vi "Shaker_DAQ.vi"() -> ()   [LabVIEW 2015]
uses:
  <vilib>/express/express analysis/Spectral/Block/exnSpectralBlock spectral measurements RMS poly.vi
  <vilib>/express/express analysis/Spectral/Block/exnSpectralBlock spectral measurements RMS DDT.vi
  <vilib>/express/express analysis/Spectral/XNode/ExpressSpectralMeasurementsBlockNode.xnode
panel:
  in  "Tab Control":T1(tab)
  in  "Test Folder":string
  in  "Input Signal":string(combo)
  in  "Date":string
  in  "PCB Type":string(combo)
  out "Beam Acceleration":dynamicdata(graph)
  out "FRF":dynamicdata(graph)
  out "FFT Magnitude":dynamicdata(graph)
  out "FFT Phase":dynamicdata(graph)
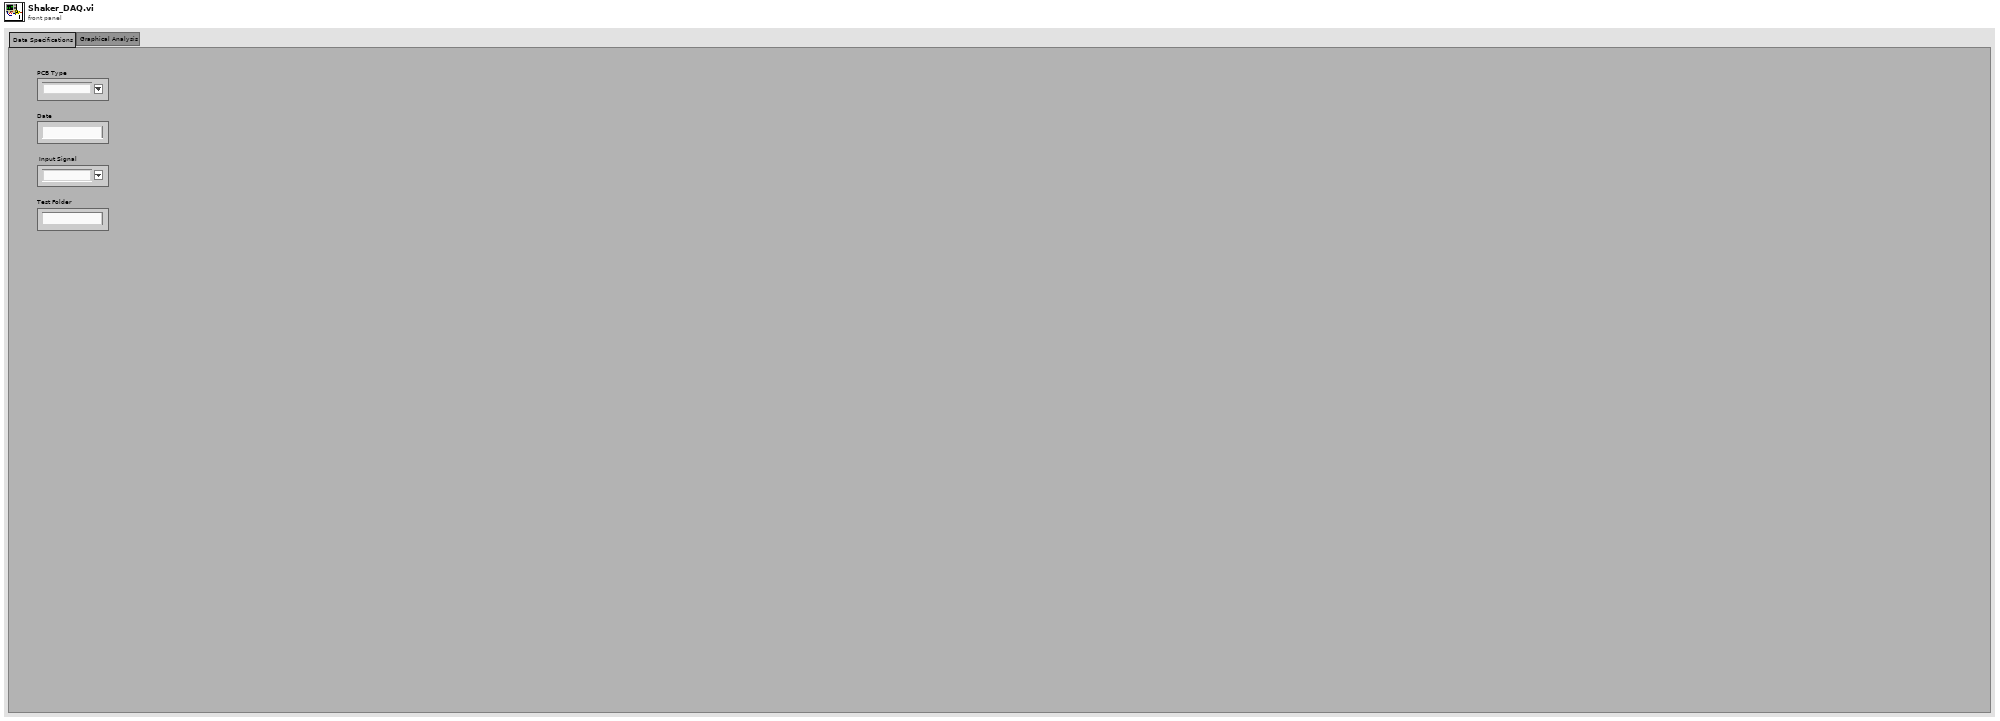
[diagram p1: front panel]
types:
  T1 = enum32{"Data Specifications", "Graphical Analysis"}
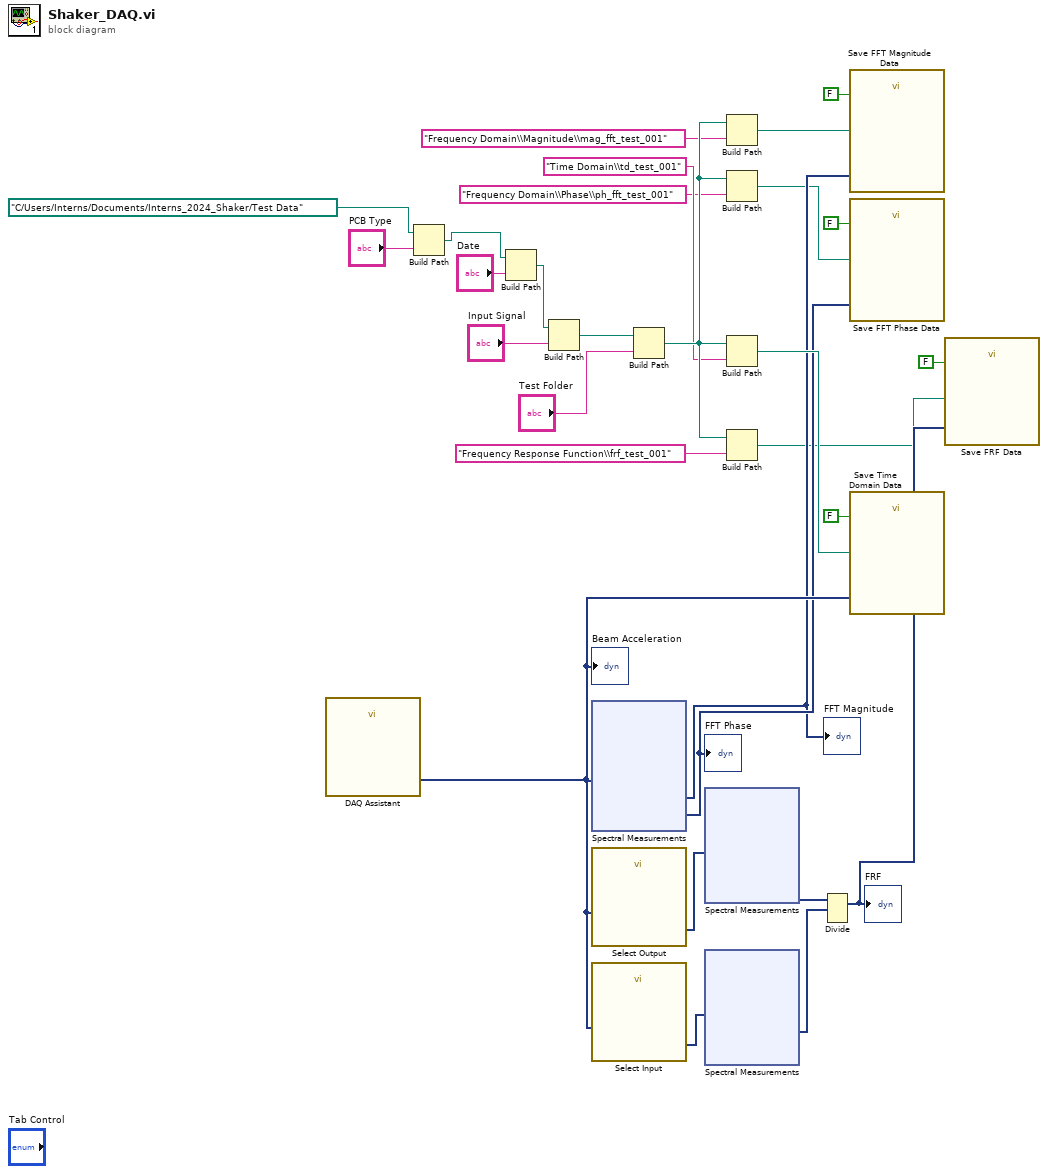
[diagram p0: block diagram]
diagram:
  n1 = call "DAQ Assistant"() -> ("data"=w10:dynamicdata)  [unwired: 17 in, 2 out]
  "Beam Acceleration" <- w10
  n2 = Build Path(base path=path "C:/Users/Interns/Documents/Interns_2024_Shaker/Test Data", name or relative path="PCB Type") -> (appended path=w24:path)
  n3 = Build Path(base path=w24, name or relative path="Date") -> (appended path=w19:path)
  n4 = Build Path(base path=w19, name or relative path="Input Signal") -> (appended path=w18:path)
  n5 = xnode "Spectral Measurements"("Signals"=w10) -> ("FFT - (RMS)"=w8:dynamicdata, "Phase"=w9:dynamicdata)  [unwired: 1 in, 1 out]
  "FFT Magnitude" <- w8
  "FFT Phase" <- w9
  n6 = call "Select Output"("Signals"=w10) -> ("Signal Out"=w26:dynamicdata)  [unwired: 9 in, 1 out]
  n7 = call "Select Input"("Signals"=w10) -> ("Signal Out"=w27:dynamicdata)  [unwired: 9 in, 1 out]
  n8 = Build Path(base path=w18, name or relative path="Test Folder") -> (appended path=w12:path)
  n9 = xnode "Spectral Measurements"("Signals"=w26) -> ("FFT - (RMS)"=w28:dynamicdata)  [unwired: 1 in, 2 out]
  n10 = xnode "Spectral Measurements"("Signals"=w27) -> ("FFT - (RMS)"=w29:dynamicdata)  [unwired: 1 in, 2 out]
  n11 = Build Path(base path=w12, name or relative path="Frequency Domain\\Magnitude\\mag_fft_test_001") -> (appended path=w3:path)
  n12 = Build Path(base path=w12, name or relative path="Frequency Domain\\Phase\\ph_fft_test_001") -> (appended path=w6:path)
  n13 = Build Path(base path=w12, name or relative path="Time Domain\\td_test_001") -> (appended path=w11:path)
  n14 = Build Path(base path=w12, name or relative path="Frequency Response Function\\frf_test_001") -> (appended path=w2:path)
  n15 = Divide(1:w29, 2:w28) -> (0:w13:dynamicdata)  [unwired: 1 in, 1 out]
  "FRF" <- w13
  n16 = call "Save FFT Magnitude Data"("Signals"=w8, "Enable"=FALSE, "Filename"=w3) -> ()  [unwired: 14 in, 3 out]
  n17 = call "Save FFT Phase Data"("Signals"=w9, "Enable"=FALSE, "Filename"=w6) -> ()  [unwired: 14 in, 3 out]
  n18 = call "Save Time Domain Data"("Signals"=w10, "Enable"=FALSE, "Filename"=w11) -> ()  [unwired: 14 in, 3 out]
  n19 = call "Save FRF Data"("Signals"=w13, "Enable"=FALSE, "Filename"=w2) -> ()  [unwired: 14 in, 3 out]
